vi "RtdeIsNewOutputDataAvailable.vi"(8 "Rtde":refnum<k24>, 11 "error in":errorcluster) -> (0 "Data available":bool, 3 "error out":errorcluster)   [LabVIEW 2020, in "UnderAutomation.UniversalRobots.lvlib"]
uses:
  UnderAutomation.UniversalRobots.lvlib
  C:/Users/fg/Documents/UniversalRobots.vi/LabVIEW_2024/UnderAutomation.UniversalRobots/lib/UnderAutomation.UniversalRobots.dll
  LabVIEW_2024/UnderAutomation.UniversalRobots/lib/UnderAutomation.UniversalRobots.dll
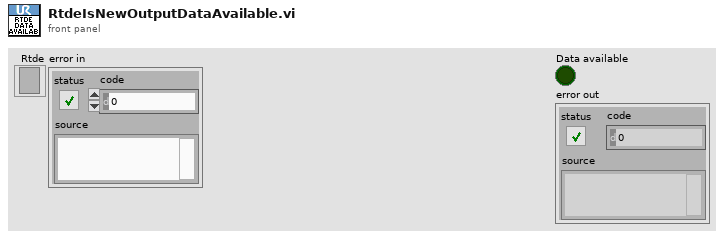
[diagram p1: front panel]
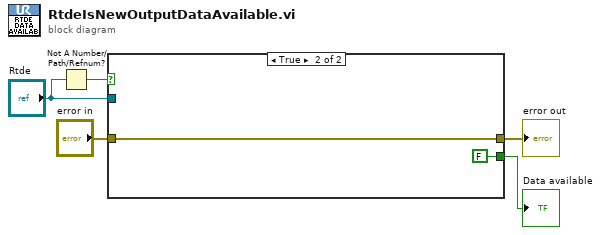
[diagram p0: block diagram]
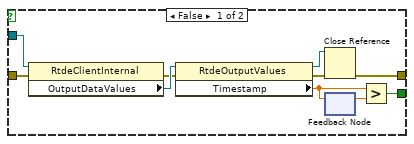
[diagram p2: hidden frame]
diagram:
  n1 = Not A Number/Path/Refnum?(number/path/refnum="Rtde") -> (NaN/Path/Refnum?=w1:bool)
  n2 = case shown="True" w1 {
    tunnel: "error in" -> [w12 w17]
    tunnel: [w10 FALSE] -> w4
    tunnel: [w7 w17] -> w3
    tunnel: "Rtde" -> [w6 _]
    frame False {
      n3 = property class="RtdeClientInternal"(reference=w6, error in=w12) -> (error out=w11:errorcluster, "OutputDataValues"=w15:refnum<k24>)  [unwired: 1 out]
      n4 = property class="RtdeOutputValues"(reference=w15, error in=w11) -> (reference out=w9:refnum<k24>, error out=w8:errorcluster, "Timestamp"=w14:dbl)
      n5 = Close Reference(reference=w9, error in (no error)=w8) -> (error out=w7:errorcluster)
      n6 = feedback #1() -> (w13:dbl)  [unwired: 1 in]
      n7 = feedback-in #1(w14) -> ()
      n8 = Greater?(x=w14, y=w13) -> (0:w10:bool)
    }
    frame True {
    }
  }
  "Data available" <- w4
  "error out" <- w3
